vi "Main.vi"() -> ()   [LabVIEW 2011]
doc: "使用该模板构建简单状态机设计模式。各状态执行代码并决定转移状态。"
uses:
  MvFGCtrlC.Net
  System.Windows.Forms
panel:
  in  "PictureBox":refnum<k24>(container) caption="图片框"
  out "cStream":refnum<k24>
  out "cDevice":refnum<k24>
  in  "正在采集":bool
  out "cSystem":refnum<k24>
  in  "关闭采集卡":bool
  in  "打开采集卡":bool
  in  "停止采集":bool
  in  "关闭相机":bool
  in  "相机列表":u16(ring)
  in  "采集卡列表":u16(ring)
  in  "cInterface":refnum<k24>
  in  "开始采集":bool
  in  "打开相机":bool
  in  "枚举相机":bool
  in  "枚举采集卡":bool
  in  "退出":bool
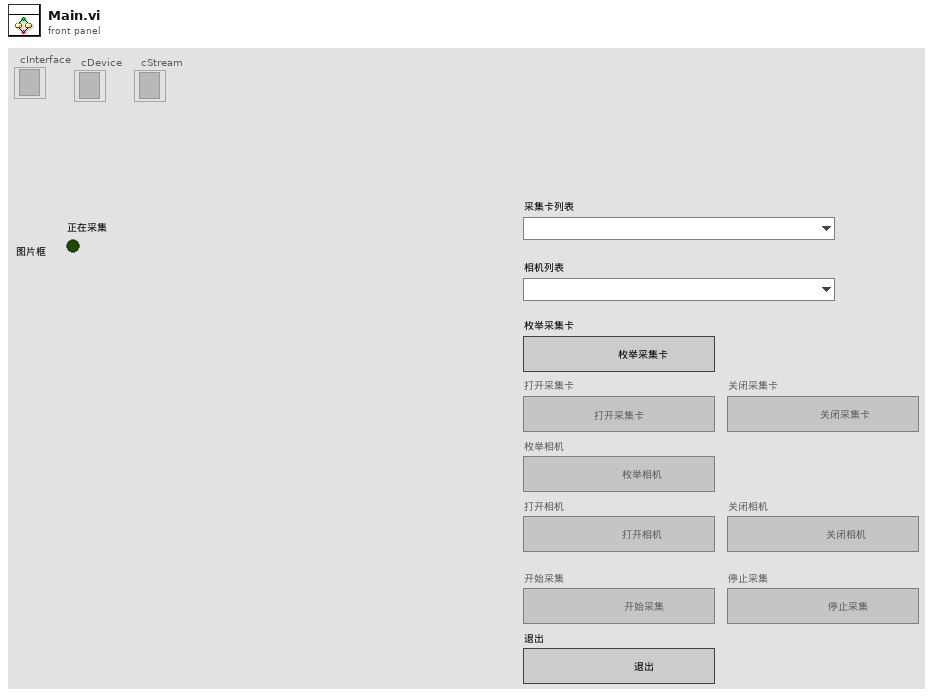
[diagram p1: front panel]
types:
  T1 = enum8{"Enabled", "Disabled", "Disabled and Grayed Out"}
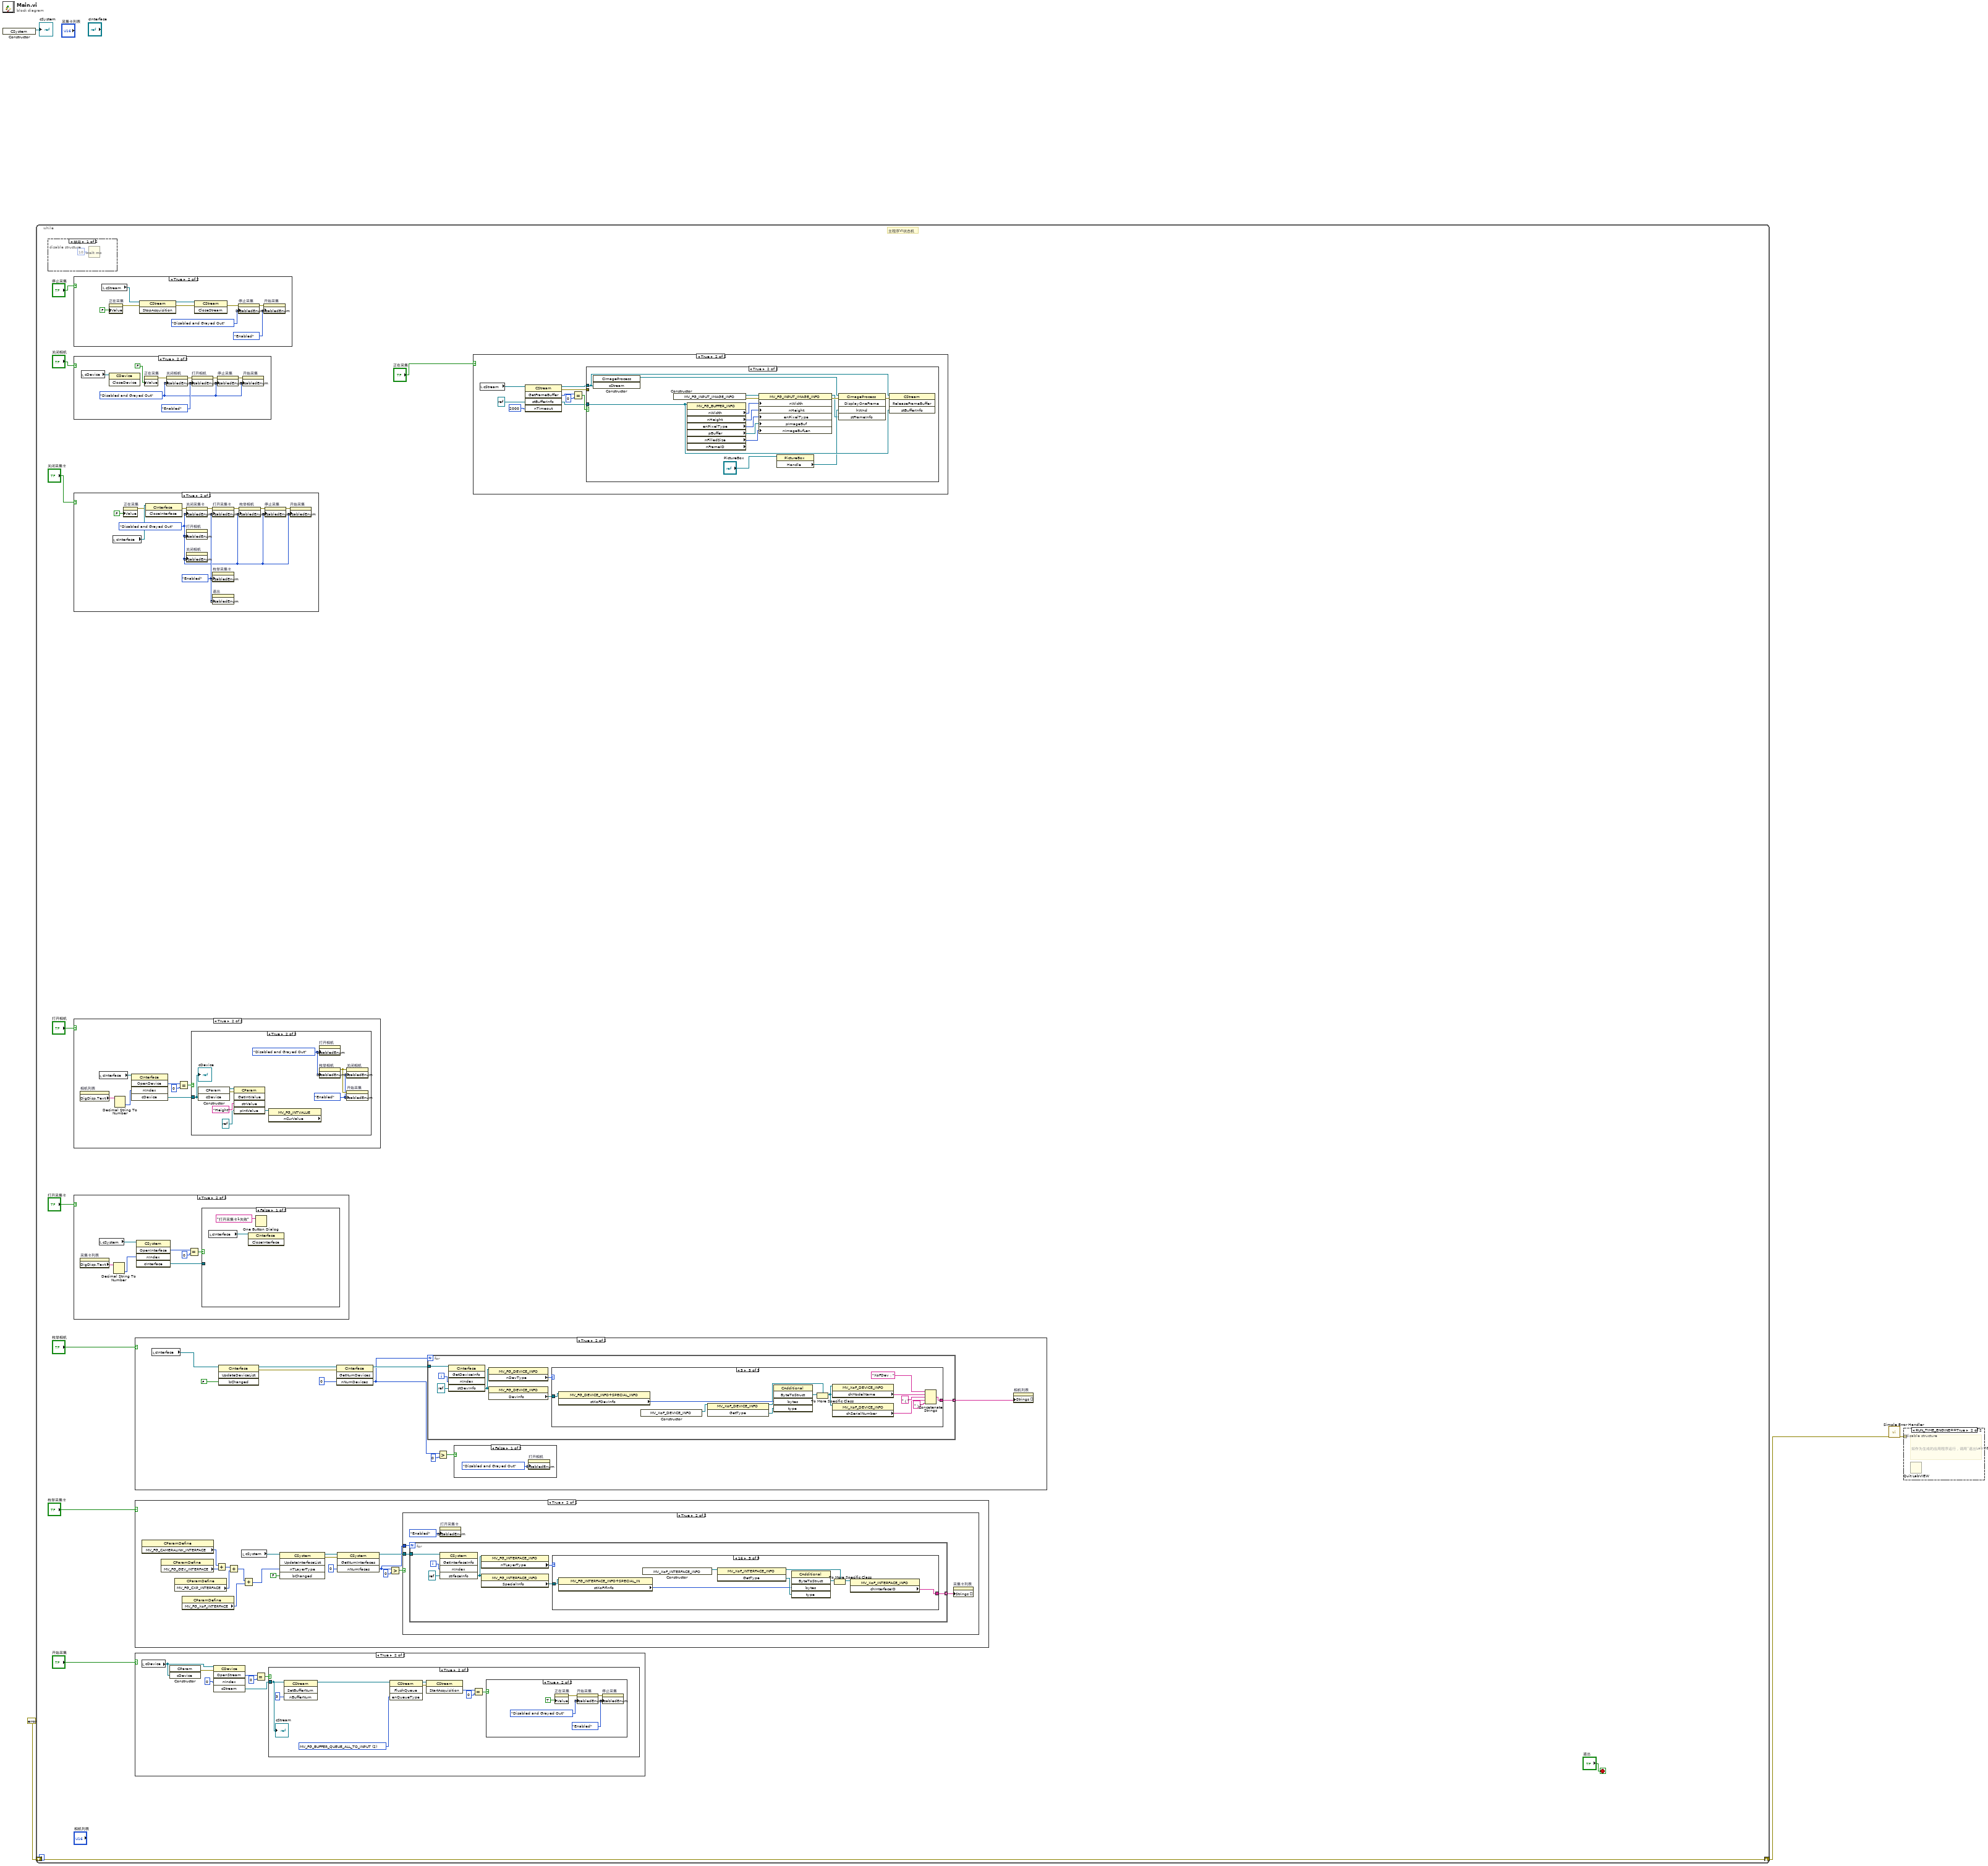
[diagram p0: block diagram]
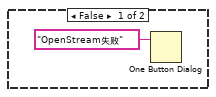
[diagram p5: hidden frame]
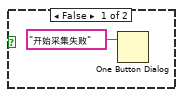
[diagram p6: hidden frame]
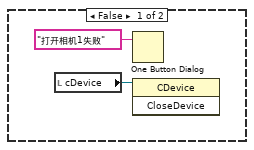
[diagram p9: hidden frame]
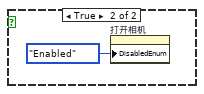
[diagram p11: hidden frame]
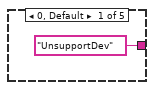
[diagram p12: hidden frame]
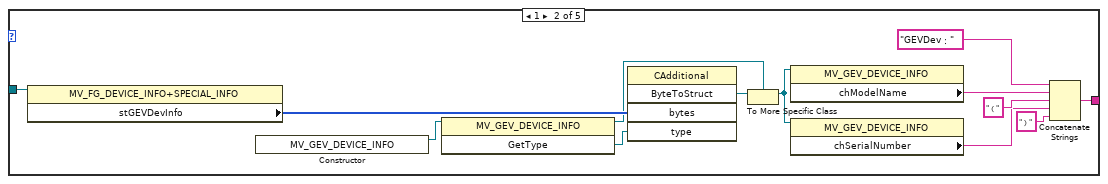
[diagram p13: hidden frame]
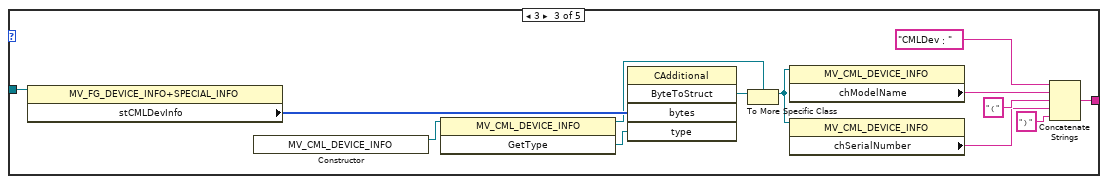
[diagram p14: hidden frame]
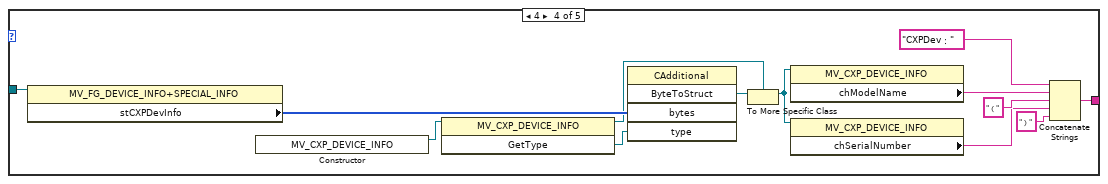
[diagram p15: hidden frame]
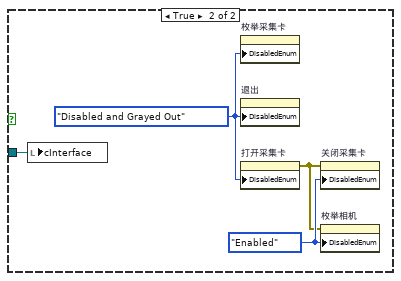
[diagram p18: hidden frame]
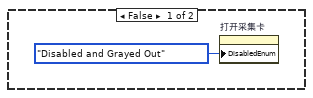
[diagram p20: hidden frame]
diagram:
  n1 = constructor class="CSystem"() -> (reference out=→"cSystem":refnum<k24>)  [unwired: 3 in, 2 out]
  n2 = while {
    shift-right: [w7] -> w3
    shift-left: errorcluster {"status"=FALSE, "code"=0, "source"=""} ("error constant") -> [w7]
    stop <- "退出" stop-if-true
    # "主程序VI状态机"
    n3 = disable-structure shown="禁用" {
      frame Disabled {
        n4 = Wait (ms)(milliseconds to wait=u32 10 ("等待时间（毫秒）")) -> ()  [unwired: 1 out]
      }
      frame Enabled {
      }
    }
    n5 = case shown="True" "停止采集" {
      frame False {
      }
      frame True {
        n6 = local read "cStream"() -> (w25:refnum<k24>)
        n7 = property on="正在采集" class="Bool (strict)"("Value"=FALSE ("正在采集")) -> (error out=w18:errorcluster)  [unwired: 2 in, 1 out]
        n8 = invoke class="CStream" method="StopAcquisition"(reference=w25, error in=w18) -> (reference out=w19:refnum<k24>, error out=w20:errorcluster)  [unwired: 1 in, 1 out]
        n9 = invoke class="CStream" method="CloseStream"(reference=w19, error in=w20) -> (error out=w17:errorcluster)  [unwired: 1 in, 2 out]
        n10 = property on="停止采集" class="Bool"(error in=w17, "DisabledEnum"=T1."Disabled and Grayed Out" ("禁用")) -> (error out=w21:errorcluster)  [unwired: 1 in, 1 out]
        n11 = property on="开始采集" class="Bool"(error in=w21, "DisabledEnum"=T1."Enabled" ("禁用")) -> ()  [unwired: 1 in, 2 out]
      }
    }
    n12 = case shown="True" "关闭相机" {
      frame False {
      }
      frame True {
        w51 = T1."Disabled and Grayed Out" ("禁用")
        n13 = local read "cDevice"() -> (w56:refnum<k24>)
        n14 = invoke on="调用节点" class="CDevice" method="CloseDevice"(reference=w56) -> ()  [unwired: 2 in, 3 out]
        n15 = property on="正在采集" class="Bool (strict)"("Value"=FALSE ("正在采集")) -> (error out=w49:errorcluster)  [unwired: 2 in, 1 out]
        n16 = property on="关闭相机" class="Bool"(error in=w49, "DisabledEnum"=w51) -> (error out=w54:errorcluster)  [unwired: 1 in, 1 out]
        n17 = property on="打开相机" class="Bool"(error in=w54, "DisabledEnum"=T1."Enabled" ("禁用")) -> (error out=w53:errorcluster)  [unwired: 1 in, 1 out]
        n18 = property on="停止采集" class="Bool"(error in=w53, "DisabledEnum"=w51) -> (error out=w52:errorcluster)  [unwired: 1 in, 1 out]
        n19 = property on="开始采集" class="Bool"(error in=w52, "DisabledEnum"=w51) -> ()  [unwired: 1 in, 2 out]
      }
    }
    n20 = case shown="True" "关闭采集卡" {
      frame False {
      }
      frame True {
        w150 = T1."Enabled" ("禁用")
        w149 = T1."Disabled and Grayed Out" ("禁用")
        n21 = local read "cInterface"() -> (w151:refnum<k24>)
        n22 = property on="正在采集" class="Bool (strict)"("Value"=FALSE ("正在采集")) -> (error out=w147:errorcluster)  [unwired: 2 in, 1 out]
        n23 = invoke on="调用节点" class="CInterface" method="CloseInterface"(reference=w151, error in=w147) -> (error out=w156:errorcluster)  [unwired: 1 in, 2 out]
        n24 = property on="关闭采集卡" class="Bool"(error in=w156, "DisabledEnum"=w149) -> (error out=w152:errorcluster)  [unwired: 1 in, 1 out]
        n25 = property on="打开相机" class="Bool"("DisabledEnum"=w149) -> ()  [unwired: 2 in, 2 out]
        n26 = property on="关闭相机" class="Bool"("DisabledEnum"=w149) -> ()  [unwired: 2 in, 2 out]
        n27 = property on="打开采集卡" class="Bool"(error in=w152, "DisabledEnum"=w150) -> (error out=w153:errorcluster)  [unwired: 1 in, 1 out]
        n28 = property on="枚举采集卡" class="Bool"("DisabledEnum"=w150) -> ()  [unwired: 2 in, 2 out]
        n29 = property on="退出" class="Bool"("DisabledEnum"=w150) -> ()  [unwired: 2 in, 2 out]
        n30 = property on="枚举相机" class="Bool"(error in=w153, "DisabledEnum"=w149) -> (error out=w154:errorcluster)  [unwired: 1 in, 1 out]
        n31 = property on="停止采集" class="Bool"(error in=w154, "DisabledEnum"=w149) -> (error out=w155:errorcluster)  [unwired: 1 in, 1 out]
        n32 = property on="开始采集" class="Bool"(error in=w155, "DisabledEnum"=w149) -> ()  [unwired: 1 in, 2 out]
      }
    }
    n33 = case shown="True" "打开相机" {
      frame False {
      }
      frame True {
        n34 = property on="相机列表" class="Ring (strict)"() -> ("DigDisp.Text"=w63:string)  [unwired: 2 in, 2 out]
        n35 = local read "cInterface"() -> (w61:refnum<k24>)
        n36 = Decimal String To Number(string=w63) -> (number=w62:i32)  [unwired: 2 in, 1 out]
        n37 = invoke on="调用节点" class="CInterface" method="OpenDevice"(reference=w61, "nIndex"=w62) -> ("OpenDevice"=w60:i32, "cDevice"=w57:refnum<k24>)  [unwired: 3 in, 3 out]
        n38 = Equal?(x=w60, y=0) -> (x = y?=w58:bool)
        n39 = case shown="True" w58 {
          tunnel: w57 -> [_ w67]
          frame False {
            n40 = local read "cDevice"() -> (w64:refnum<k24>)
            n41 = One Button Dialog(message="打开相机1失败" ("消息")) -> ()  [unwired: 1 in, 1 out]
            n42 = invoke on="调用节点" class="CDevice" method="CloseDevice"(reference=w64) -> ()  [unwired: 2 in, 3 out]
          }
          frame True {
            w66 = T1."Enabled" ("禁用")
            w73 = T1."Disabled and Grayed Out" ("禁用")
            n43 = constructor class="CParam"("cDevice"=w67) -> (reference out=w71:refnum<k24>, error out=w72:errorcluster)  [unwired: 3 in, 2 out]
            n44 = invoke class="CParam" method="GetIntValue"(reference=w71, error in=w72, "strValue"="Height", "pIntValue"=refnum<k24> refnum) -> ("pIntValue"=w69:refnum<k24>)  [unwired: 1 in, 4 out]
            n45 = property class="MV_FG_INTVALUE" props=["nCurValue"](reference=w69) -> ()  [unwired: 1 in, 3 out]
            n46 = property on="打开相机" class="Bool"("DisabledEnum"=w73) -> ()  [unwired: 2 in, 2 out]
            n47 = property on="枚举相机" class="Bool"("DisabledEnum"=w73) -> (error out=w74:errorcluster)  [unwired: 2 in, 1 out]
            n48 = property on="关闭相机" class="Bool"(error in=w74, "DisabledEnum"=w66) -> ()  [unwired: 1 in, 2 out]
            n49 = property on="开始采集" class="Bool"(error in=w74, "DisabledEnum"=w66) -> ()  [unwired: 1 in, 2 out]
            "cDevice" <- w67
          }
        }
      }
    }
    n50 = case shown="True" "打开采集卡" {
      frame False {
      }
      frame True {
        n51 = property on="采集卡列表" class="Ring (strict)"() -> ("DigDisp.Text"=w162:string)  [unwired: 2 in, 2 out]
        n52 = local read "cSystem"() -> (w163:refnum<k24>)
        n53 = Decimal String To Number(string=w162) -> (number=w161:i32)  [unwired: 2 in, 1 out]
        n54 = invoke on="调用节点" class="CSystem" method="OpenInterface"(reference=w163, "nIndex"=w161) -> ("OpenInterface"=w159:i32, "cInterface"=w160:refnum<k24>)  [unwired: 3 in, 3 out]
        n55 = Equal?(x=w159, y=0) -> (x = y?=w157:bool)
        n56 = case shown="False" w157 {
          tunnel: w160 -> [_ w169]
          frame False {
            n57 = local read "cInterface"() -> (w164:refnum<k24>)
            n58 = invoke on="调用节点" class="CInterface" method="CloseInterface"(reference=w164) -> ()  [unwired: 2 in, 3 out]
            n59 = One Button Dialog(message="打开采集卡1失败" ("消息")) -> ()  [unwired: 1 in, 1 out]
          }
          frame True {
            w168 = T1."Enabled" ("禁用")
            w166 = T1."Disabled and Grayed Out" ("禁用")
            n60 = local write "cInterface"(w169) -> ()
            n61 = property on="枚举采集卡" class="Bool"("DisabledEnum"=w166) -> ()  [unwired: 2 in, 2 out]
            n62 = property on="退出" class="Bool"("DisabledEnum"=w166) -> ()  [unwired: 2 in, 2 out]
            n63 = property on="打开采集卡" class="Bool"("DisabledEnum"=w166) -> (error out=w167:errorcluster)  [unwired: 2 in, 1 out]
            n64 = property on="关闭采集卡" class="Bool"(error in=w167, "DisabledEnum"=w168) -> ()  [unwired: 1 in, 2 out]
            n65 = property on="枚举相机" class="Bool"(error in=w167, "DisabledEnum"=w168) -> ()  [unwired: 1 in, 2 out]
          }
        }
      }
    }
    n66 = case shown="True" "枚举相机" {
      frame False {
      }
      frame True {
        n67 = local read "cInterface"() -> (w75:refnum<k24>)
        n68 = invoke on="调用节点" class="CInterface" method="UpdateDeviceList"(reference=w75, "bChanged"=FALSE) -> (reference out=w80:refnum<k24>, error out=w79:errorcluster)  [unwired: 2 in, 2 out]
        n69 = invoke on="调用节点" class="CInterface" method="GetNumDevices"(reference=w80, error in=w79, "nNumDevices"=u32 0) -> (reference out=w82:refnum<k24>, "nNumDevices"=w78:u32)  [unwired: 1 in, 2 out]
        n70 = for {
          N: w78 -> [_]
          tunnel: w82 -> [w92]
          tunnel: [w88] -> w84 mode=indexing
          i -> [w93]
          n71 = invoke class="CInterface" method="GetDeviceInfo"(reference=w92, "nIndex"=w93, "stDevInfo"=refnum<k24> refnum) -> ("stDevInfo"=w91:refnum<k24>)  [unwired: 2 in, 4 out]
          n72 = property class="MV_FG_DEVICE_INFO"(reference=w91) -> ("nDevType"=w90:u32)  [unwired: 1 in, 2 out]
          n73 = property class="MV_FG_DEVICE_INFO"(reference=w91) -> ("DevInfo"=w89:refnum<k24>)  [unwired: 1 in, 2 out]
          n74 = case shown="5" w90 {
            tunnel: w89 -> [_ w107 w108 w121 w135]
            tunnel: ["UnsupportDev" w97 w109 w122 w134] -> w88
            frame 0, Default {
            }
            frame 1 {
              n75 = property class="MV_FG_DEVICE_INFO+SPECIAL_INFO"(reference=w107) -> ("stGEVDevInfo"=w106:u8[])  [unwired: 1 in, 2 out]
              n76 = constructor class="MV_GEV_DEVICE_INFO"() -> (reference out=w105:refnum<k24>)  [unwired: 3 in, 2 out]
              n77 = invoke on="调用节点" class="MV_GEV_DEVICE_INFO" method="GetType"(reference=w105) -> (reference out=w102:refnum<k24>, "GetType"=w104:refnum<k24>)  [unwired: 2 in, 1 out]
              n78 = invoke on="调用节点" class="CAdditional" method="ByteToStruct"("bytes"=w106, "type"=w104) -> ("ByteToStruct"=w103:refnum<k24>)  [unwired: 3 in, 4 out]
              n79 = To More Specific Class(target class=w102, reference=w103) -> (specific class reference=w98:refnum<k24>)  [unwired: 1 in, 1 out]
              n80 = property class="MV_GEV_DEVICE_INFO"(reference=w98) -> ("chModelName"=w96:string)  [unwired: 1 in, 2 out]
              n81 = property class="MV_GEV_DEVICE_INFO"(reference=w98) -> ("chSerialNumber"=w99:string)  [unwired: 1 in, 2 out]
              n82 = Concatenate Strings("GEVDev：" ("字符串"), w96, "（" ("字符串"), w99, "）" ("字符串")) -> (w97:string)
            }
            frame 3 {
              n83 = property class="MV_FG_DEVICE_INFO+SPECIAL_INFO"(reference=w108) -> ("stCMLDevInfo"=w120:u8[])  [unwired: 1 in, 2 out]
              n84 = constructor class="MV_CML_DEVICE_INFO"() -> (reference out=w119:refnum<k24>)  [unwired: 3 in, 2 out]
              n85 = invoke on="调用节点" class="MV_CML_DEVICE_INFO" method="GetType"(reference=w119) -> (reference out=w116:refnum<k24>, "GetType"=w118:refnum<k24>)  [unwired: 2 in, 1 out]
              n86 = invoke on="调用节点" class="CAdditional" method="ByteToStruct"("bytes"=w120, "type"=w118) -> ("ByteToStruct"=w117:refnum<k24>)  [unwired: 3 in, 4 out]
              n87 = To More Specific Class(target class=w116, reference=w117) -> (specific class reference=w112:refnum<k24>)  [unwired: 1 in, 1 out]
              n88 = property class="MV_CML_DEVICE_INFO"(reference=w112) -> ("chModelName"=w111:string)  [unwired: 1 in, 2 out]
              n89 = property class="MV_CML_DEVICE_INFO"(reference=w112) -> ("chSerialNumber"=w113:string)  [unwired: 1 in, 2 out]
              n90 = Concatenate Strings("CMLDev：" ("字符串"), w111, "（" ("字符串"), w113, "）" ("字符串")) -> (w109:string)
            }
            frame 4 {
              n91 = property class="MV_FG_DEVICE_INFO+SPECIAL_INFO"(reference=w121) -> ("stCXPDevInfo"=w133:u8[])  [unwired: 1 in, 2 out]
              n92 = constructor class="MV_CXP_DEVICE_INFO"() -> (reference out=w132:refnum<k24>)  [unwired: 3 in, 2 out]
              n93 = invoke on="调用节点" class="MV_CXP_DEVICE_INFO" method="GetType"(reference=w132) -> (reference out=w129:refnum<k24>, "GetType"=w131:refnum<k24>)  [unwired: 2 in, 1 out]
              n94 = invoke on="调用节点" class="CAdditional" method="ByteToStruct"("bytes"=w133, "type"=w131) -> ("ByteToStruct"=w130:refnum<k24>)  [unwired: 3 in, 4 out]
              n95 = To More Specific Class(target class=w129, reference=w130) -> (specific class reference=w125:refnum<k24>)  [unwired: 1 in, 1 out]
              n96 = property class="MV_CXP_DEVICE_INFO"(reference=w125) -> ("chModelName"=w124:string)  [unwired: 1 in, 2 out]
              n97 = property class="MV_CXP_DEVICE_INFO"(reference=w125) -> ("chSerialNumber"=w126:string)  [unwired: 1 in, 2 out]
              n98 = Concatenate Strings("CXPDev：" ("字符串"), w124, "（" ("字符串"), w126, "）" ("字符串")) -> (w122:string)
            }
            frame 5 {
              n99 = property class="MV_FG_DEVICE_INFO+SPECIAL_INFO"(reference=w135) -> ("stXoFDevInfo"=w146:u8[])  [unwired: 1 in, 2 out]
              n100 = constructor class="MV_XoF_DEVICE_INFO"() -> (reference out=w145:refnum<k24>)  [unwired: 3 in, 2 out]
              n101 = invoke on="调用节点" class="MV_XoF_DEVICE_INFO" method="GetType"(reference=w145) -> (reference out=w142:refnum<k24>, "GetType"=w144:refnum<k24>)  [unwired: 2 in, 1 out]
              n102 = invoke on="调用节点" class="CAdditional" method="ByteToStruct"("bytes"=w146, "type"=w144) -> ("ByteToStruct"=w143:refnum<k24>)  [unwired: 3 in, 4 out]
              n103 = To More Specific Class(target class=w142, reference=w143) -> (specific class reference=w138:refnum<k24>)  [unwired: 1 in, 1 out]
              n104 = property class="MV_XoF_DEVICE_INFO"(reference=w138) -> ("chModelName"=w137:string)  [unwired: 1 in, 2 out]
              n105 = property class="MV_XoF_DEVICE_INFO"(reference=w138) -> ("chSerialNumber"=w139:string)  [unwired: 1 in, 2 out]
              n106 = Concatenate Strings("XoFDev：" ("字符串"), w137, "（" ("字符串"), w139, "）" ("字符串")) -> (w134:string)
            }
          }
        }
        n107 = Greater?(x=w78, y=u32 0) -> (0:w76:bool)
        n108 = case shown="False" w76 {
          frame False {
            n109 = property on="打开相机" class="Bool"("DisabledEnum"=T1."Disabled and Grayed Out" ("禁用")) -> ()  [unwired: 2 in, 2 out]
          }
          frame True {
            n110 = property on="打开相机" class="Bool"("DisabledEnum"=T1."Enabled" ("禁用")) -> ()  [unwired: 2 in, 2 out]
          }
        }
        n111 = property on="相机列表" class="Ring (strict)"("Strings []"=w84) -> ()  [unwired: 2 in, 2 out]
      }
    }
    n112 = case shown="True" "枚举采集卡" {
      frame False {
      }
      frame True {
        n113 = property class="CParamDefine"() -> ("MV_FG_CAMERALINK_INTERFACE"=w184:i32)  [unwired: 2 in, 2 out]
        n114 = property class="CParamDefine"() -> ("MV_FG_GEV_INTERFACE"=w183:i32)  [unwired: 2 in, 2 out]
        n115 = property class="CParamDefine"() -> ("MV_FG_CXP_INTERFACE"=w175:i32)  [unwired: 2 in, 2 out]
        n116 = property class="CParamDefine"() -> ("MV_FG_XoF_INTERFACE"=w172:i32)  [unwired: 2 in, 2 out]
        n117 = Add(x=w184, y=w183) -> (x+y=w176:i32)
        n118 = Add(x=w176, y=w175) -> (x+y=w171:i32)
        n119 = local read "cSystem"() -> (w173:refnum<k24>)
        n120 = Add(x=w171, y=w172) -> (x+y=w170:i32)
        n121 = invoke on="调用节点" class="CSystem" method="UpdateInterfaceList"(reference=w173, "nTLayerType"=w170, "bChanged"=FALSE) -> (reference out=w177:refnum<k24>, error out=w180:errorcluster)  [unwired: 2 in, 3 out]
        n122 = invoke class="CSystem" method="GetNumInterfaces"(reference=w177, error in=w180, "nNumIfaces"=u32 0) -> (reference out=w178:refnum<k24>, "nNumIfaces"=w174:u32)  [unwired: 1 in, 2 out]
        n123 = Greater?(x=w174, y=u32 0) -> (0:w179:bool)
        n124 = case shown="True" w179 {
          tunnel: w178 -> [_ w190]
          tunnel: w174 -> [_ w188]
          frame False {
            n125 = property on="打开采集卡" class="Bool"("DisabledEnum"=T1."Disabled and Grayed Out" ("禁用")) -> ()  [unwired: 2 in, 2 out]
          }
          frame True {
            n126 = for {
              N: w188 -> [_]
              tunnel: w190 -> [w197]
              tunnel: [w194] -> w187 mode=indexing
              i -> [w196]
              n127 = invoke class="CSystem" method="GetInterfaceInfo"(reference=w197, "nIndex"=w196, "stIfaceInfo"=refnum<k24> refnum) -> ("stIfaceInfo"=w193:refnum<k24>)  [unwired: 2 in, 4 out]
              n128 = property class="MV_FG_INTERFACE_INFO"(reference=w193) -> ("nTLayerType"=w191:u32)  [unwired: 1 in, 2 out]
              n129 = property class="MV_FG_INTERFACE_INFO"(reference=w193) -> ("SpecialInfo"=w192:refnum<k24>)  [unwired: 1 in, 2 out]
              n130 = case shown="16" w191 {
                tunnel: ["" ("chInterfaceID") w200 w207 w215 w224] -> w194
                tunnel: w192 -> [_ w205 w208 w216 w223]
                frame Default {
                }
                frame 1 {
                  n131 = property class="MV_FG_INTERFACE_INFO+SPECIAL_IN"(reference=w205) -> ("stGevIfInfo"=w206:u8[])  [unwired: 1 in, 2 out]
                  n132 = constructor class="MV_GEV_INTERFACE_INFO"() -> (reference out=w204:refnum<k24>)  [unwired: 3 in, 2 out]
                  n133 = invoke on="调用节点" class="MV_GEV_INTERFACE_INFO" method="GetType"(reference=w204) -> (reference out=w201:refnum<k24>, "GetType"=w199:refnum<k24>)  [unwired: 2 in, 1 out]
                  n134 = invoke on="调用节点" class="CAdditional" method="ByteToStruct"("bytes"=w206, "type"=w199) -> ("ByteToStruct"=w203:refnum<k24>)  [unwired: 3 in, 4 out]
                  n135 = To More Specific Class(target class=w201, reference=w203) -> (specific class reference=w202:refnum<k24>)  [unwired: 1 in, 1 out]
                  n136 = property class="MV_GEV_INTERFACE_INFO"(reference=w202) -> ("chInterfaceID"=w200:string)  [unwired: 1 in, 2 out]
                }
                frame 4 {
                  n137 = property class="MV_FG_INTERFACE_INFO+SPECIAL_IN"(reference=w208) -> ("stCMLIfInfo"=w214:u8[])  [unwired: 1 in, 2 out]
                  n138 = constructor class="MV_CML_INTERFACE_INFO"() -> (reference out=w213:refnum<k24>)  [unwired: 3 in, 2 out]
                  n139 = invoke on="调用节点" class="MV_CML_INTERFACE_INFO" method="GetType"(reference=w213) -> (reference out=w210:refnum<k24>, "GetType"=w209:refnum<k24>)  [unwired: 2 in, 1 out]
                  n140 = invoke on="调用节点" class="CAdditional" method="ByteToStruct"("bytes"=w214, "type"=w209) -> ("ByteToStruct"=w212:refnum<k24>)  [unwired: 3 in, 4 out]
                  n141 = To More Specific Class(target class=w210, reference=w212) -> (specific class reference=w211:refnum<k24>)  [unwired: 1 in, 1 out]
                  n142 = property class="MV_CML_INTERFACE_INFO"(reference=w211) -> ("chInterfaceID"=w207:string)  [unwired: 1 in, 2 out]
                }
                frame 8 {
                  n143 = property class="MV_FG_INTERFACE_INFO+SPECIAL_IN"(reference=w216) -> ("stCXPIfInfo"=w222:u8[])  [unwired: 1 in, 2 out]
                  n144 = constructor class="MV_CXP_INTERFACE_INFO"() -> (reference out=w221:refnum<k24>)  [unwired: 3 in, 2 out]
                  n145 = invoke on="调用节点" class="MV_CXP_INTERFACE_INFO" method="GetType"(reference=w221) -> (reference out=w218:refnum<k24>, "GetType"=w217:refnum<k24>)  [unwired: 2 in, 1 out]
                  n146 = invoke on="调用节点" class="CAdditional" method="ByteToStruct"("bytes"=w222, "type"=w217) -> ("ByteToStruct"=w220:refnum<k24>)  [unwired: 3 in, 4 out]
                  n147 = To More Specific Class(target class=w218, reference=w220) -> (specific class reference=w219:refnum<k24>)  [unwired: 1 in, 1 out]
                  n148 = property class="MV_CXP_INTERFACE_INFO"(reference=w219) -> ("chInterfaceID"=w215:string)  [unwired: 1 in, 2 out]
                }
                frame 16 {
                  n149 = property class="MV_FG_INTERFACE_INFO+SPECIAL_IN"(reference=w223) -> ("stXoFIfInfo"=w225:u8[])  [unwired: 1 in, 2 out]
                  n150 = constructor class="MV_XoF_INTERFACE_INFO"() -> (reference out=w226:refnum<k24>)  [unwired: 3 in, 2 out]
                  n151 = invoke on="调用节点" class="MV_XoF_INTERFACE_INFO" method="GetType"(reference=w226) -> (reference out=w229:refnum<k24>, "GetType"=w230:refnum<k24>)  [unwired: 2 in, 1 out]
                  n152 = invoke on="调用节点" class="CAdditional" method="ByteToStruct"("bytes"=w225, "type"=w230) -> ("ByteToStruct"=w227:refnum<k24>)  [unwired: 3 in, 4 out]
                  n153 = To More Specific Class(target class=w229, reference=w227) -> (specific class reference=w228:refnum<k24>)  [unwired: 1 in, 1 out]
                  n154 = property class="MV_XoF_INTERFACE_INFO"(reference=w228) -> ("chInterfaceID"=w224:string)  [unwired: 1 in, 2 out]
                }
              }
            }
            n155 = property on="打开采集卡" class="Bool"("DisabledEnum"=T1."Enabled" ("禁用")) -> ()  [unwired: 2 in, 2 out]
            n156 = property on="采集卡列表" class="Ring (strict)"("Strings []"=w187) -> ()  [unwired: 2 in, 2 out]
          }
        }
      }
    }
    n157 = case shown="True" "开始采集" {
      frame False {
      }
      frame True {
        n158 = local read "cDevice"() -> (w27:refnum<k24>)
        n159 = constructor class="CParam"("cDevice"=w27) -> (error out=w26:errorcluster)  [unwired: 3 in, 3 out]
        n160 = invoke on="调用节点" class="CDevice" method="OpenStream"(reference=w27, error in=w26, "nIndex"=u32 0) -> ("OpenStream"=w30:i32, "cStream"=w32:refnum<k24>)  [unwired: 2 in, 3 out]
        n161 = Equal?(x=w30, y=0) -> (x = y?=w28:bool)
        n162 = case shown="True" w28 {
          tunnel: w32 -> [_ w36]
          frame False {
            n163 = One Button Dialog(message="OpenStream失败" ("消息")) -> ()  [unwired: 1 in, 1 out]
          }
          frame True {
            w35 = 2 items=["MV_FG_BUFFER_QUEUE_INPUT_TO_OUTPUT", "MV_FG_BUFFER_QUEUE_OUTPUT_DISCARD", "MV_FG_BUFFER_QUEUE_ALL_TO_INPUT", "MV_FG_BUFFER_QUEUE_UNQUEUED_TO_INPUT", "MV_FG_BUFFER_QUEUE_ALL_DISCARD"] ("enQueueType")
            n164 = invoke on="调用节点" class="CStream" method="SetBufferNum"(reference=w36, "nBufferNum"=u32 3) -> (reference out=w34:refnum<k24>)  [unwired: 2 in, 3 out]
            n165 = invoke on="调用节点" class="CStream" method="FlushQueue"(reference=w34, "enQueueType"=w35) -> (reference out=w42:refnum<k24>, error out=w41:errorcluster)  [unwired: 2 in, 2 out]
            n166 = invoke on="调用节点" class="CStream" method="StartAcquisition"(reference=w42, error in=w41) -> ("StartAcquisition"=w40:i32)  [unwired: 1 in, 2 out]
            n167 = Equal?(x=w40, y=0) -> (x = y?=w38:bool)
            n168 = case shown="True" w38 {
              frame False {
                n169 = One Button Dialog(message="开始采集失败" ("消息")) -> ()  [unwired: 1 in, 1 out]
              }
              frame True {
                n170 = property on="正在采集" class="Bool (strict)"("Value"=TRUE ("正在采集")) -> (error out=w44:errorcluster)  [unwired: 2 in, 1 out]
                n171 = property on="开始采集" class="Bool"(error in=w44, "DisabledEnum"=T1."Disabled and Grayed Out" ("禁用")) -> (error out=w48:errorcluster)  [unwired: 1 in, 1 out]
                n172 = property on="停止采集" class="Bool"(error in=w48, "DisabledEnum"=T1."Enabled" ("禁用")) -> ()  [unwired: 1 in, 2 out]
              }
            }
            "cStream" <- w36
          }
        }
      }
    }
    n173 = case shown="True" "正在采集" {
      frame False {
      }
      frame True {
        n174 = local read "cStream"() -> (w236:refnum<k24>)
        n175 = invoke class="CStream" method="GetFrameBuffer"(reference=w236, "stBufferInfo"=refnum<k24> refnum, "nTimeout"=u32 2000) -> (reference out=w232:refnum<k24>, error out=w231:errorcluster, "GetFrameBuffer"=w239:i32, "stBufferInfo"=w233:refnum<k24>)  [unwired: 2 in, 1 out]
        n176 = Equal?(x=w239, y=0) -> (x = y?=w237:bool)
        n177 = case shown="True" w237 {
          tunnel: w233 -> [_ w252]
          tunnel: w232 -> [_ w247]
          tunnel: w231 -> [_ _]
          frame False {
          }
          frame True {
            n178 = constructor class="CImageProcess"("cStream"=w247) -> (reference out=w254:refnum<k24>)  [unwired: 3 in, 3 out]
            n179 = constructor class="MV_FG_INPUT_IMAGE_INFO"() -> (reference out=w241:refnum<k24>, error out=w240:errorcluster)  [unwired: 3 in, 1 out]
            n180 = property class="MV_FG_BUFFER_INFO" props=["nWidth", "nHeight", "enPixelType", "pBuffer", "nFilledSize", "nFrameID"](reference=w252) -> ("nWidth"=w251:u32, "nHeight"=w250:u32, "enPixelType"=w249:i32, "pBuffer"=w248:refnum<k24>, "nFilledSize"=w246:u32)  [unwired: 1 in, 3 out]
            n181 = property class="MV_FG_INPUT_IMAGE_INFO"(reference=w241, error in=w240, "nWidth"=w251, "nHeight"=w250, "enPixelType"=w249, "pImageBuf"=w248, "nImageBufLen"=w246) -> (reference out=w242:refnum<k24>, error out=w243:errorcluster)
            n182 = property class="PictureBox"(reference="PictureBox") -> ("Handle"=w244:refnum<k24>)  [unwired: 1 in, 2 out]
            n183 = invoke class="CImageProcess" method="DisplayOneFrame"(reference=w254, error in=w243, "hWnd"=w244, "stFrameInfo"=w242) -> (error out=w253:errorcluster)  [unwired: 1 in, 4 out]
            n184 = invoke class="CStream" method="ReleaseFrameBuffer"(reference=w247, error in=w253, "stBufferInfo"=w252) -> ()  [unwired: 1 in, 4 out]
          }
        }
      }
    }
  }
  n185 = call <vilib>:"Simple Error Handler.vi"("error in (no error)"=w3) -> ("error out"=w2:errorcluster)  [unwired: 4 in, 4 out]
  n186 = disable-structure shown="RUN_TIME_ENGINE==True" {
    disable-tunnel: w2 -> [_ _]
    frame condition #0 (active) {
    }
    frame condition #1 {
      # "如作为生成的应用程序运行，调用“退出LabVIEW”。"
      n187 = Quit LabVIEW() -> ()  [unwired: 1 in]
    }
  }
